vi "snapAndEnqueueImages.vi"(8 "queue in":refnum<queue>, 9 "user event in":refnum<user-event>, 11 "Session In":T1) -> ()   [LabVIEW 2013]
uses:
  <vilib>/userdefined/High Color/IMAQdx.ctl
  <vilib>/vision/driver/NI_Vision_Acquisition_Software.lvlib
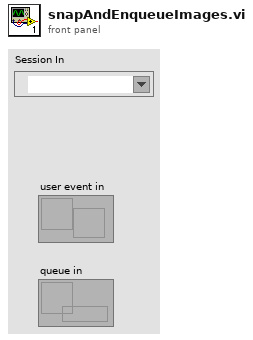
[diagram p1: front panel]
types:
  T1 = typedef "IMAQdx.ctl" = refnum<k21>
  T2 = typedef "IMAQ Image.ctl" = refnum<image>
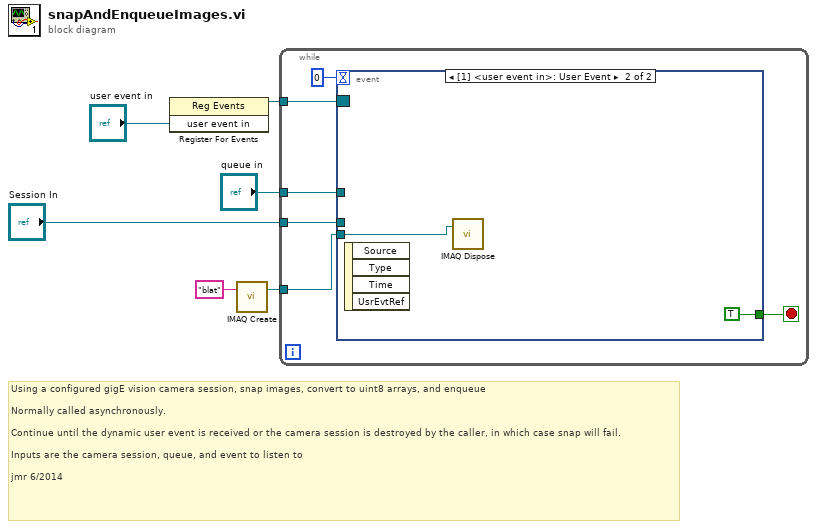
[diagram p0: block diagram]
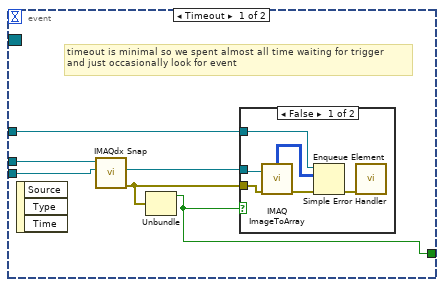
[diagram p2: hidden frame]
diagram:
  # "Using a configured gigE vision camera session, snap images, convert to uint8 arrays, and enqueue\n\nNormally called asynchronously.  \n\nContinue until the dynamic user event is received or the camera session is destroyed by the caller, in which case snap will fail.\n\nInputs are the camera session, queue, and event to listen to\n\njmr 6/2014"
  n1 = register-events("user event in") -> (reference out=w3:refnum<event-registration>)  [unwired: 2 in, 1 out]
  n2 = call "IMAQ Create"("Image Name"="blat") -> ("New Image"=w2:T2)  [unwired: 4 in, 1 out]
  n3 = while {
    tunnel: "queue in" -> [w8]
    tunnel: w3 -> [w11]
    tunnel: w2 -> [w9]
    tunnel: "Session In" -> [w7]
    stop <- w10 stop-if-true
    n4 = event shown="[1] <user event in>: User Event" {
      selector: w11 -> [_ _]
      dyn-events: _ -> [_ _]
      timeout: 0 -> [_ _]
      tunnel: [w13 TRUE] -> w10
      tunnel: w9 -> [w17 w25]
      tunnel: w8 -> [w16 _]
      tunnel: w7 -> [w15 _]
      event Timeout {
        # "timeout is minimal so we spent almost all time waiting for trigger\nand just occasionally look for event"
        n5 = event-data() -> ()  [unwired: 1 in, 3 out]
        n6 = call <vilib>:"IMAQdx Snap.vi"("Image In"=w17, "Session In"=w15) -> ("error out"=w14:errorcluster, "Image Out"=w18:T2)  [unwired: 7 in, 1 out]
        n7 = Unbundle(w14) -> ("status"=w13:bool)  [unwired: 2 out]
        n8 = case shown="False" w13 {
          tunnel: w18 -> [w20 _]
          tunnel: w16 -> [w21 _]
          tunnel: w14 -> [w19 _]
          frame False {
            n9 = call "IMAQ ImageToArray"("error in (no error)"=w19, "Image"=w20) -> ("error out"=w23:errorcluster, "Image Pixels (U8)"=w22:u8[][])  [unwired: 2 in, 3 out]
            n10 = Enqueue Element(queue=w21, element=w22, error in (no error)=w23) -> (error out=w24:errorcluster)  [unwired: 1 in, 2 out]
            n11 = call <vilib>:"Simple Error Handler.vi"("error in (no error)"=w24) -> ()  [unwired: 4 in, 5 out]
          }
          frame True {
          }
        }
      }
      event User Event {
        n12 = event-data() -> ()  [unwired: 1 in, 4 out]
        n13 = call "IMAQ Dispose"("Image"=w25) -> ()  [unwired: 5 in, 1 out]
      }
    }
  }
